vi "Replace Factory.vi"(8 "error in (no error)":errorcluster, 10 "Field Factory":refnum<class "Column Factory.lvclass">, 11 "Basic Table in":refnum<class "Basic Table.lvclass">) -> (0 "error out":errorcluster, 3 "Basic Table out":refnum<class "Basic Table.lvclass">)   [LabVIEW 2020, in "Table.lvlib" / "Basic Table.lvclass"]
uses:
  Basic Table.lvclass
  Column Libraries/Basic Columns/Column Configuration/Column Factory Parent Class/Column Factory.lvclass
  Basic Table.lvclass/Basic Table.ctl
  Table Configuration Interface/Table Configuration Interface.lvclass
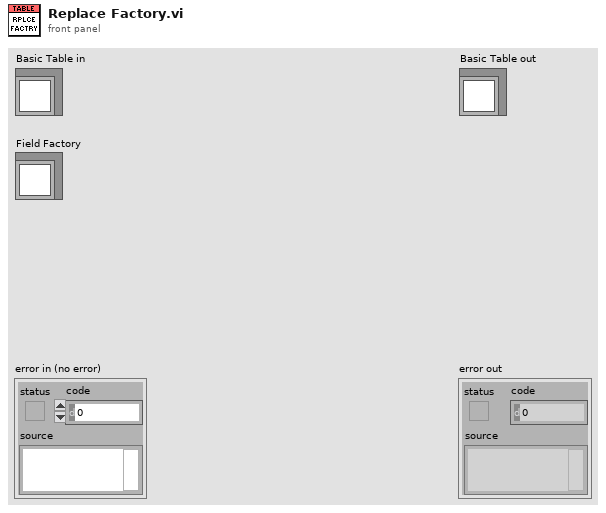
[diagram p1: front panel]
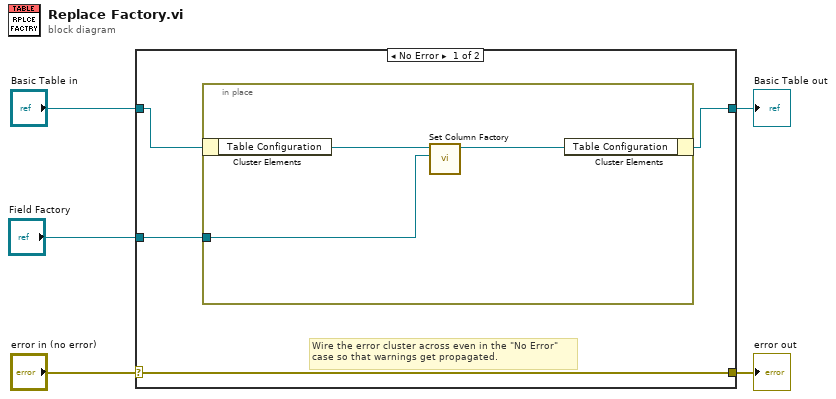
[diagram p0: block diagram]
diagram:
  n1 = case shown="No Error" "error in (no error)" {
    selector: "error in (no error)" -> [w9 w14]
    tunnel: [w9 w14] -> w4
    tunnel: [w6 w13] -> w2
    tunnel: "Basic Table in" -> [w8 w13]
    tunnel: "Field Factory" -> [w7 _]
    frame No Error {
      # "Wire the error cluster across even in the \"No Error\"\ncase so that warnings get propagated."
      n2 = in-place {
        in-place-border: w7 -> [w11]
        n3 = in-place-cluster #1(w8) -> ("Table Configuration"=w12:refnum<class "Table Configuration Interface.lvclass">)
        n4 = call-dynamic "Set Column Factory.vi"("Column Factory Type"=w11, "Table Configuration Interface in"=w12) -> ("Table Configuration Interface out"=w10:refnum<class "Table Configuration Interface.lvclass">)  [unwired: 8 in, 1 out]
        n5 = in-place-cluster #1("Table Configuration"=w10) -> (w6:refnum<class "Basic Table.lvclass">)
      }
    }
    frame Error {
    }
  }
  "error out" <- w4
  "Basic Table out" <- w2
